vi "_OLS_RunReport_Rev3.vi"() -> ()   [LabVIEW 2024]
uses:
  Control Definitions/Def Results2.ctl
  Control Definitions/Def_ATPStatus.ctl
  Control Definitions/Def_PumpSpeed.ctl
  Control Definitions/Def TestState.ctl
  Control Definitions/DEF_CalConstants.ctl
  Control Definitions/Def PumpCtlRefs.ctl
  Control Definitions/Def CalTable.ctl
  Control Definitions/Def CalCoef.ctl
  Control Definitions/Def_LevelCalCoef.ctl
  Control Definitions/Registry Keys.ctl
  Control Definitions/Global 2.vi
  Control Definitions/Global 1.vi
panel:
  in  "Get File Data":bool=TRUE
  in  "Level PV":dbl(slide)=8.0 scale=8.5..2.0
  out "File Name":string
  out "Root path":path
  out "Numeric":i32
  out "Cal Coef":T1={"Level"={"M"=-0.9990777034816695, "B"=9.617362923679963, "Mc"=-1.0009231479344565, "Bc"=9.626241172397878, "LMe"=7.844}, "Dataq Ch"=[{"B"=-0.34241100677002123, "M"=175.4094780519764}, {"B"=-0.7865736704446391, "M"=174.89102005231038}]}
  in  "Default Cal Table":T3={"Level"={"LSf"=2.6, "LMf"=3.511, "LKf"=6.112, "LMe"=7.844, "LKe"=1.775, "LSe"=8.0}, "DataQ CH"=[{"RqLA"=0.577, "RmLA"=102.9, "RqHA"=5.052, "RmHA"=904.4}, {"RqLA"=0.577, "RmLA"=101.1, "RqHA"=5.116, "RmHA"=903.4}]}
  out "ItemPath":string
  in  "End Prog":bool=TRUE
  out "Test Index Out":i32
  out "PumpCtlRef out":T4
  out "Reg Cal Constants":T5={"Measure High"="", "Laser High"="", "Measure Low"="", "Laser Low"="", "Cal Name"="", "Cal Date"="9/24/2024 9:21:12 AM", "Empty Inches"=8.0, "Full Inches"=2.6, "Valid"=FALSE}
  in  "Skip Pre-Lube":bool=TRUE
  out "TEST State Out":T6
  in  "Pump Speed":T7
  out "Ch B  Sim":dbl=101.0
  out "Ch A  Sim":dbl=200.0
  out "Root Path":path=path "C:/AllenProjects/PWC-OLS"
  out "Time(ms)":dbl=1249.4499999994114
  out "Level":bool=TRUE
  out "DataQ":bool=TRUE
  in  "Check":bool
  out "Laser (raw)":dbl=1.9040000438690186 format="%#_4g"
  out "Results out":T8 {"Resistor" format="%.1f"; "Drain" format="%.3f"; "Fill" format="%.3f"}
  in  "DUT":i16=1
  in  "Pump JOG":bool=TRUE
  in  "Run Test":bool
  in  "Normal":cluster{u32, u32}[](array[cluster])=[{16711680, 1244948}]
  in  "Sim Color":cluster{u32, u32}[](array[cluster])=[{16774656, 1244948}]
  out "Level \nStatus":bool=TRUE
  out "DataQ\nStatus":bool=TRUE
  in  "Level SP":dbl(slide)=8.0 scale=8.5..2.0
  out "Level":dbl=7.715118932422306 format="%.3f"
  in  "Drain":bool
  in  "Fill":bool
  in  "Simulate":bool
  out "TEST NME":string="OLR001--cal"
  out "DataQ Input":T10(graph)={"ChA Ohms"=100.83065830421491, "ChB Ohms"=100.0340857774357, "Laser (raw)"=1.9040000438690186}
  out "Time Stamp":timestamp=timestamp(3810639016.2712703 s since 1904-01-01)
  in  "stop":bool
  out "ChB Ohms":dbl=100.0340857774357 format="%.1f"
  out "ChA Ohms":dbl=100.79497115454612 format="%.1f"
  out "TimeBase":dbl=100.79497115454612 format="%.1f"
  # "Calibration & Scaling Table\n               Tank         Key          Ref\n               Scale        Level        Measure\nEmpty\n\n\nFull"
  # "8.0      1.7752      7.844\n\n2.6      6.112        3.511"
  # "CHA"
  # "CHB"
  # "ATP       Resistance     Fill        Drain"
  # "ATP       Resistance     Fill        Drain"
  # "Simulated Resistor In"
  # "PUMP"
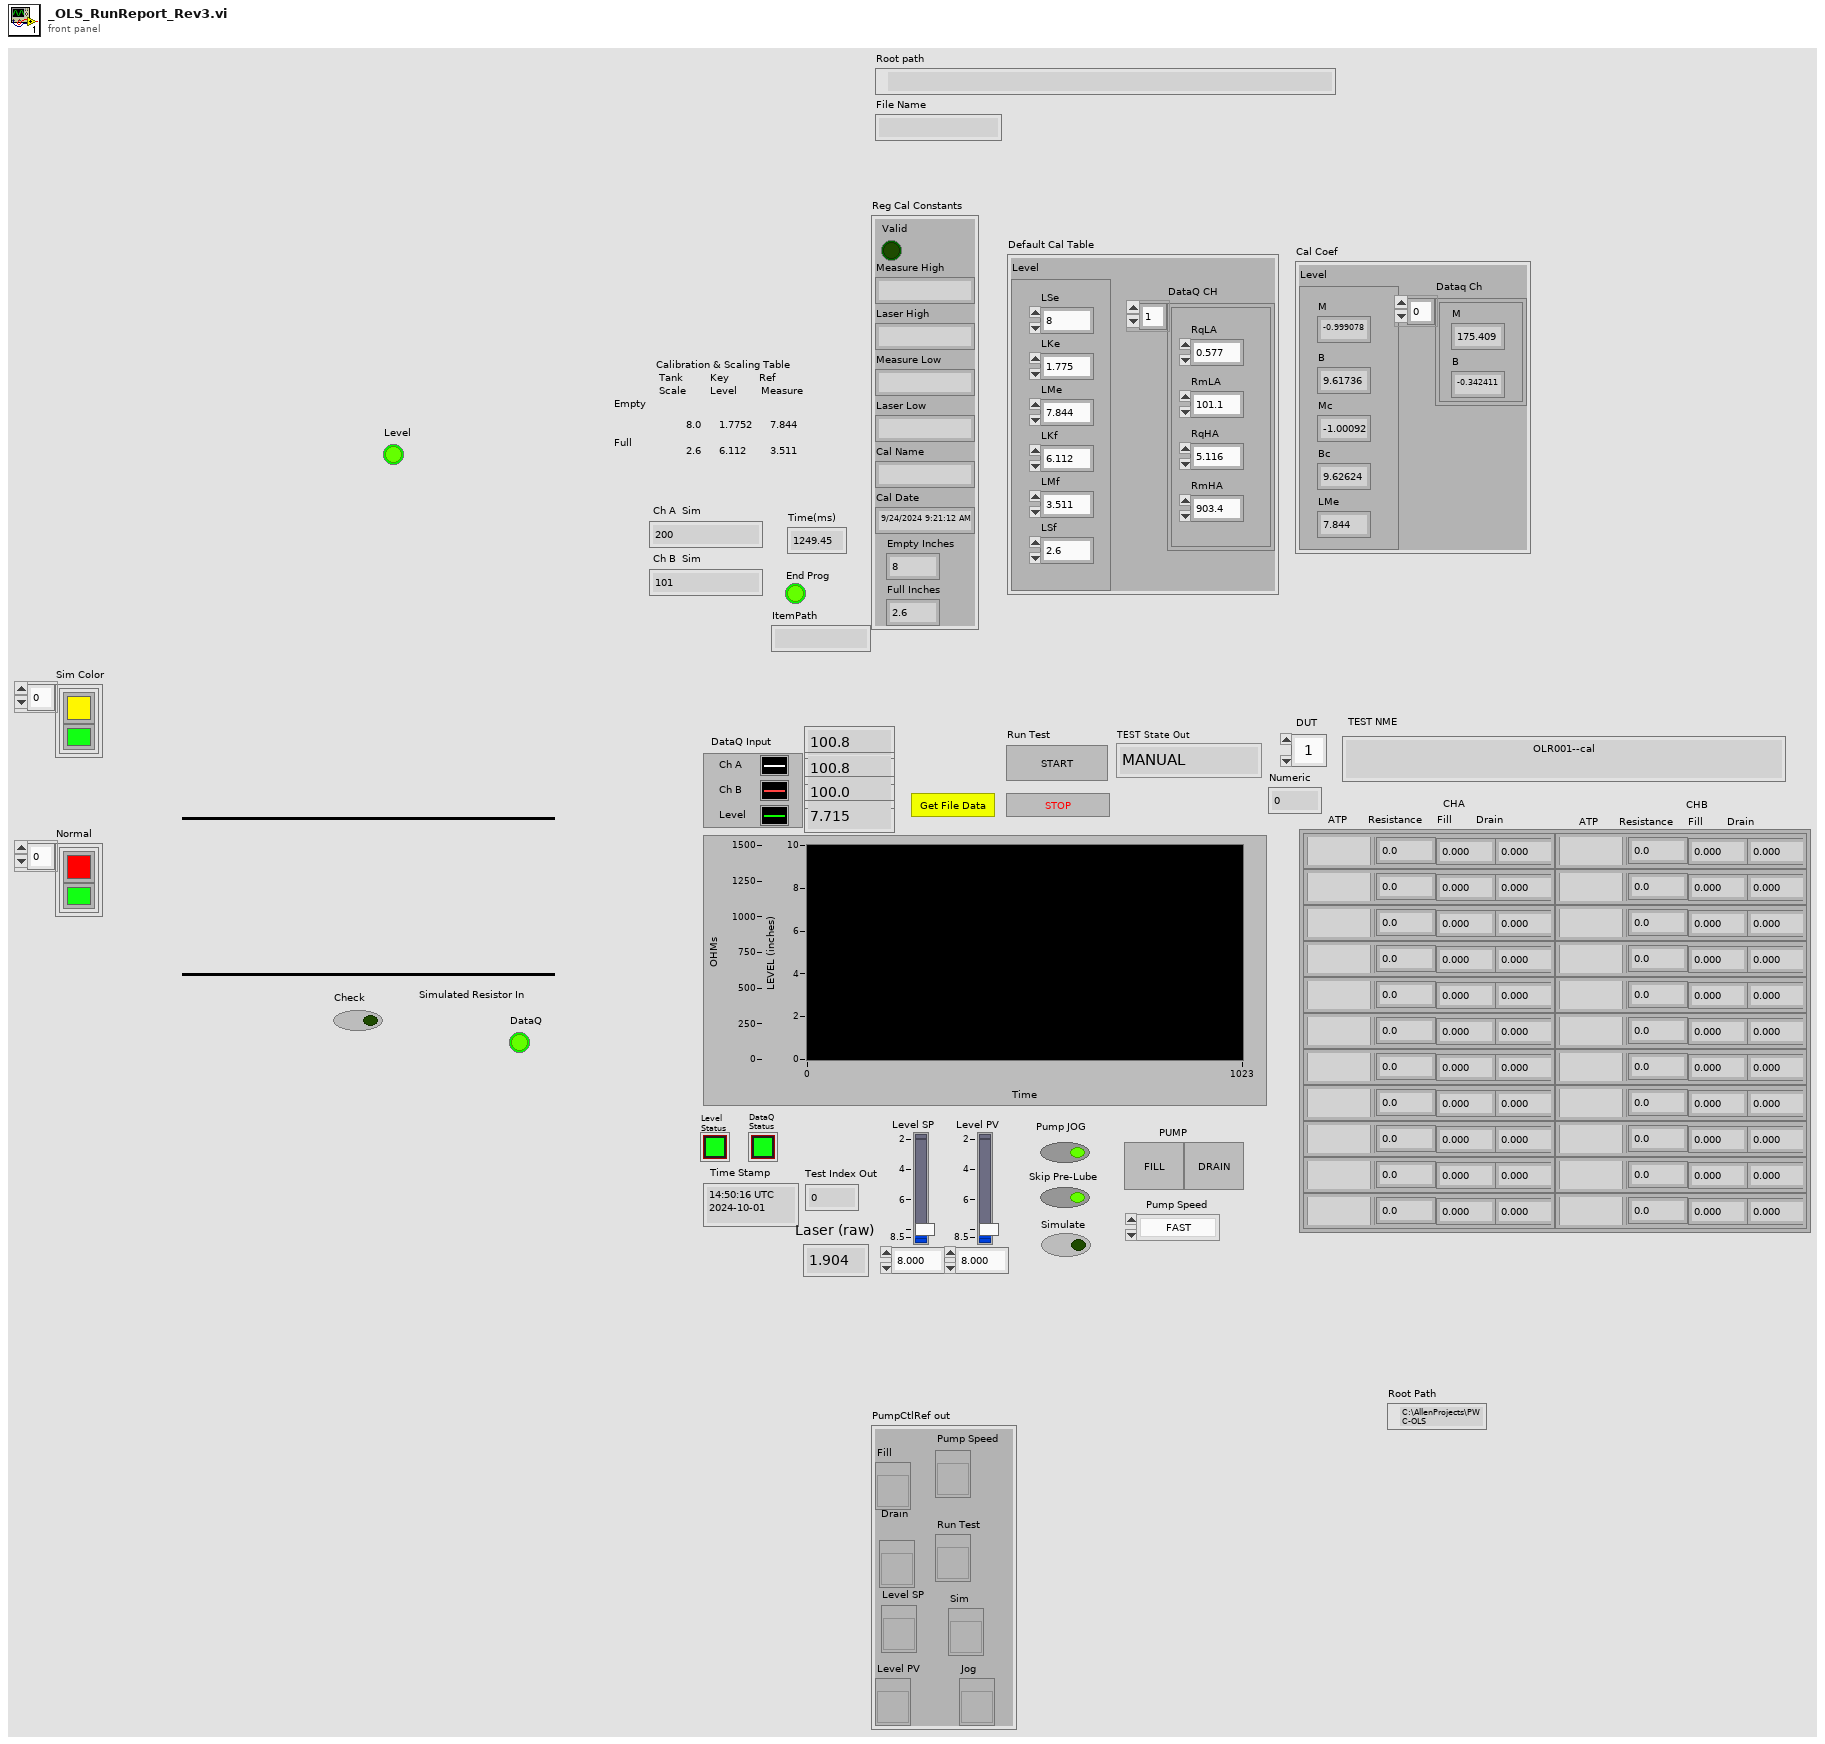
[diagram p1: front panel]
types:
  T1 = typedef "Def CalCoef.ctl" = cluster{"Level":T2, "Dataq Ch":cluster{"B":dbl, "M":dbl}[]}
  T2 = typedef "Def_LevelCalCoef.ctl" = cluster{"M":dbl, "B":dbl, "Mc":dbl, "Bc":dbl, "LMe":dbl}
  T3 = typedef "Def CalTable.ctl" = cluster{"Level":cluster{"LSf":dbl, "LMf":dbl, "LKf":dbl, "LMe":dbl, "LKe":dbl, "LSe":dbl}, "DataQ CH":cluster{"RqLA":dbl, "RmLA":dbl, "RqHA":dbl, "RmHA":dbl}[]}
  T4 = typedef "Def PumpCtlRefs.ctl" = cluster{"Fill ":refnum<vi>, "Drain":refnum<vi>, "Level PV":refnum<vi>, "Pump Speed":refnum<vi>, "Run Test":refnum<vi>, "Sim":refnum<vi>, "Jog":refnum<vi>, "Level SP":refnum<vi>}
  T5 = typedef "DEF_CalConstants.ctl" = cluster{"Measure High":string, "Laser High":string, "Measure Low":string, "Laser Low":string, "Cal Name":string, "Cal Date":string, "Empty Inches":dbl, "Full Inches":dbl, "Valid":bool}
  T6 = typedef "Def TestState.ctl" = enum16{"MANUAL", "Start", "Pre-Fill", "Pre-Fill Measure", "Pre-Drain", "Pre-Drin Measure", "Init-Record", "Load Fill Spec", "Filling Hi", "Wait1", "Record Fill", "Load Drain Spec", "Draining Lo", "Wait2", "Record Drain", "Empty", "Done"}
  T7 = typedef "Def_PumpSpeed.ctl" = enum16{"FAST", "SLOW", "CREEP", "STOP"}
  T8 = typedef "Def Results2.ctl" = cluster{"Fill":dbl, "Drain":dbl, "Status":T9, "Resistor":dbl}[][]
  T9 = typedef "Def_ATPStatus.ctl" = i16
  T10 = cluster{"ChA Ohms":dbl, "ChB Ohms":dbl, "Laser (raw)":dbl}
  T11 = typedef "Registry Keys.ctl" = enum16{"Report Files Key", "Config Files Key"}
  T12 = cluster{"Level \nStatus":refnum<vi>, "DataQ\nStatus":refnum<vi>}
  T13 = typedef "Def FullCfg.ctl" = cluster{"Bench Config":T14, "Test Value Table ":dbl[][], "Table Col Titles":string[][], "cluster":T4, "Bench Status":T15}
  T14 = typedef "Def BenchCfg.ctl" = cluster{"Name":string, cluster{"Step Levels":dbl, "Tolerance":dbl, "Sample Rate":dbl, "Resistor":dbl, "M Level Cal":dbl, "[B Level Cal":dbl, "Max Fill Rate":dbl, "Empty Inches":dbl, "Full Inches":dbl}}
  T15 = typedef "Def Bench Status.ctl" = cluster{"Pump Status":refnum<vi>, "Instrumnet\n Status":refnum<vi>}
  T16 = enum16{"MANUAL", "Start", "Filling", "FULL", "Draining", "EMPTY", "Done"}
  T17 = cluster{"Resistor":dbl, "Fill":dbl, "Drain":dbl, "Status":i16}
  T18 = cluster{"Resistor":dbl, "Fill":dbl, "Drain":dbl, "Status":i16}[][]
  T19 = typedef "DEF_SpecsOut.ctl" = cluster{"aSpecsTable":T20[], "Pump CtlRef In":T4, "TEST State Out":T6, "TEST Index":i32, "Drain!Fill":bool}
  T20 = typedef "Def Spec RNG.ctl" = cluster{"Specs":dbl[], "LUT Status":T21}
  T21 = typedef "Ded LUT_Status.ctl" = cluster{"ChA/!ChB":bool, "Drain/!Fill":bool, "In Range?":bool, "Switch Range?":bool, "Measure R?":bool, "Vaild R?":bool, "Index(n)":i32, "Index(n)-1":i32, "Index Max":i32, "Index(n-1)":i32}
  T22 = typedef "Def Measure.ctl" = cluster{"ChA R":dbl, "ChB R":dbl, "Level PV":dbl}
  T23 = cluster{"Resistor":dbl, "Fill":dbl, "Drain":dbl, "Resistor":dbl}[][]
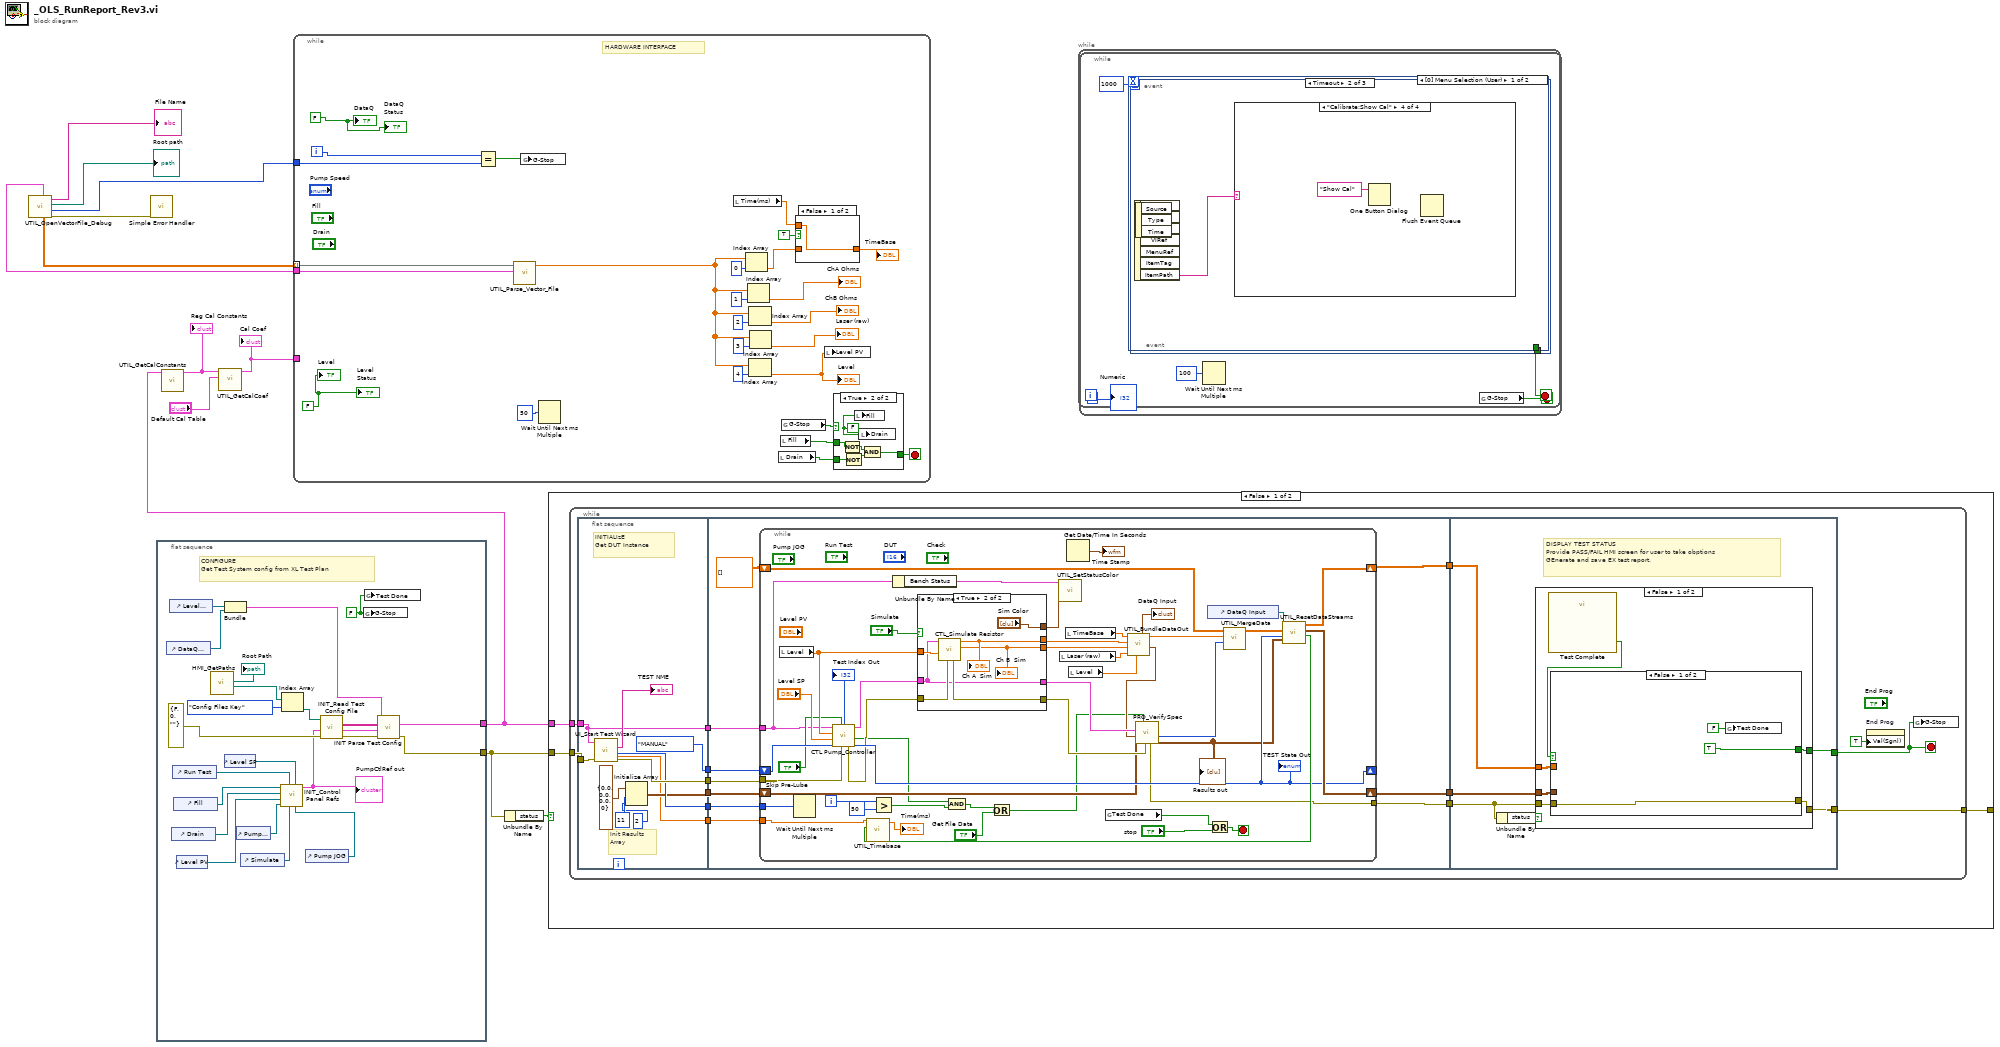
[diagram p0: block diagram]
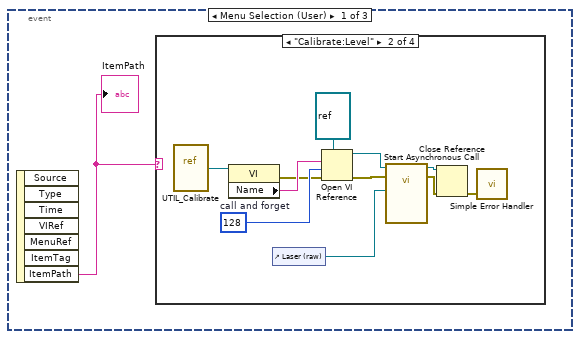
[diagram p2: hidden frame]
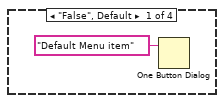
[diagram p3: hidden frame]
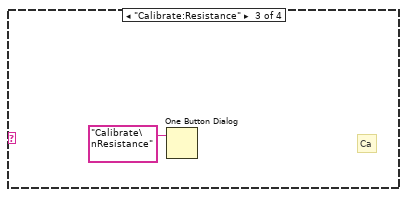
[diagram p4: hidden frame]
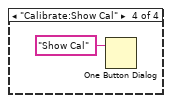
[diagram p5: hidden frame]
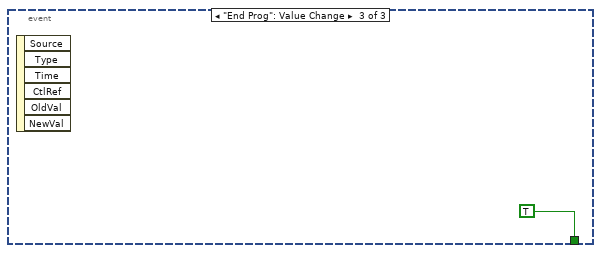
[diagram p6: hidden frame]
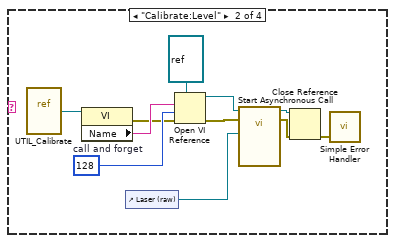
[diagram p8: hidden frame]
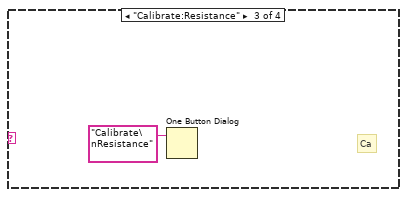
[diagram p9: hidden frame]
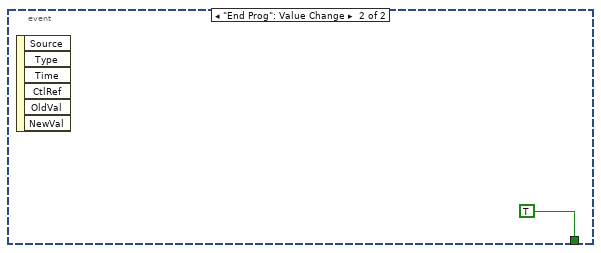
[diagram p10: hidden frame]
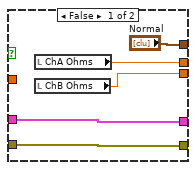
[diagram p11: hidden frame]
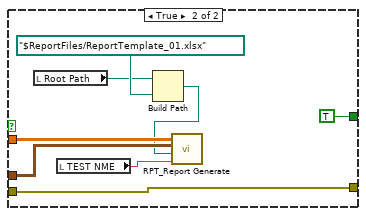
[diagram p12: hidden frame]
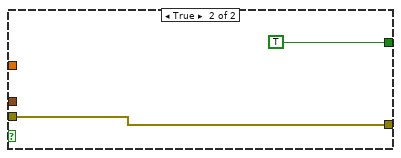
[diagram p13: hidden frame]
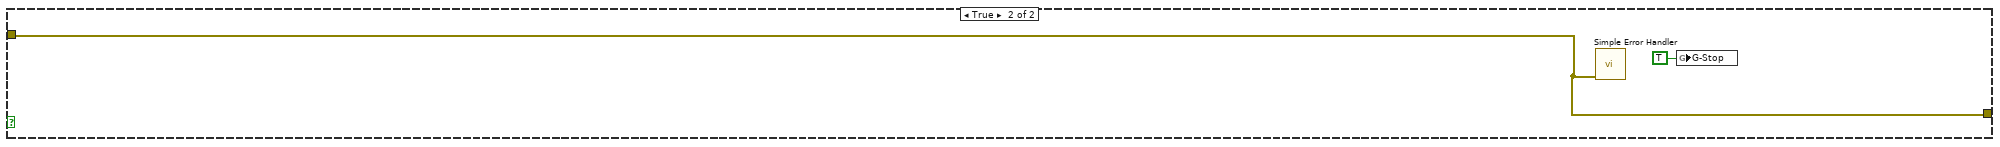
[diagram p14: hidden frame]
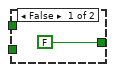
[diagram p16: hidden frame]
diagram:
  n1 = call "UTIL_OpenVectorFile_Debug.vi"() -> ("error out"=w4:errorcluster, "Count"=w1:i32, "path"=→"Root path":path, "File Name"=→"File Name":string, "Data"=w3:dbl[][], "Cal Coef Out"=w2:T1)  [unwired: 6 in]
  n2 = call <vilib>:"Simple Error Handler.vi"("error in (no error)"=w4) -> ()  [unwired: 4 in, 5 out]
  n3 = flat-sequence {
    tunnel: [w32] -> w11
    tunnel: [w25] -> w9
    frame #0 {
      w20 = FALSE ("G-Stop")
      # "CONFIGURE\nGet Test System config from XL Test Plan"
      n4 = control-ref of="DataQ\nStatus"() -> (w22:refnum<vi>)
      n5 = control-ref of="Level \nStatus"() -> (w31:refnum<vi>)
      n6 = control-ref of="Drain"() -> (w33:refnum<vi>)
      n7 = control-ref of="Run Test"() -> (w27:refnum<vi>)
      n8 = control-ref of="Fill"() -> (w28:refnum<vi>)
      n9 = control-ref of="Level PV"() -> (w13:refnum<vi>)
      n10 = call "HMI_GetPaths.vi"() -> ("Default Paths"=w15:path[], "Root Path"=→"Root Path":path)  [unwired: 10 in]
      n11 = Bundle("Level \nStatus"=w31, "DataQ\nStatus"=w22) -> (w30:T12)  [unwired: 1 in]
      n12 = control-ref of="Level SP"() -> (w21:refnum<vi>)
      n13 = control-ref of="Pump Speed"() -> (w17:refnum<vi>)
      n14 = control-ref of="Simulate"() -> (w24:refnum<vi>)
      n15 = Index Array(array=w15, index=Registry_Keys."Config Files Key" ("Reg Key")) -> (element=w14:path)
      n16 = control-ref of="Pump JOG"() -> (w23:refnum<vi>)
      n17 = call "INIT_Control Panel Refs.vi"("Jog"=w23, "Level SP"=w21, "Sim"=w24, "Run Test"=w27, "Pump Speed"=w17, "Level PV"=w13, "Drain"=w33, "Fill"=w28) -> ("PumpCtlRef out"=w18:T4)  [unwired: 3 in]
      "PumpCtlRef out" <- w18
      n18 = call "INIT_Read Test Config File.vi"("error in (no error)"=errorcluster {"status"=FALSE, "code"=0, "source"=""}, "Path"=w14) -> ("error out 2"=w26:errorcluster, "Config\nFile Data"=w29:string[][])  [unwired: 8 in]
      n19 = global write "Global 1.vi" "G-Stop"(w20) -> ()
      n20 = global write "Global 2.vi" "Test Done"(w20) -> ()
      n21 = call "INIT Parse Test Config.vi"("error in (no error)"=w26, "Pump CtlRef In"=w18, "All XL Input"=w29, "Bench Status"=w30) -> ("error out"=w32:errorcluster, "Full Config"=w25:T13)  [unwired: 5 in, 1 out]
    }
  }
  n22 = call "UTIL_GetCalConstants.vi"("Full Config"=w9) -> ("Cal Constants"=w10:T5)  [unwired: 9 in, 1 out]
  "Reg Cal Constants" <- w10
  n23 = call "UTIL_GetCalCoef.vi"("Cal Table"="Default Cal Table", "Cal Constants"=w10) -> ("Cal Coef"=w7:T1)  [unwired: 9 in]
  "Cal Coef" <- w7
  n24 = while {
    tunnel: w7 -> [_]
    tunnel: w3 -> [w55] mode=indexing
    tunnel: w2 -> [w49]
    tunnel: w1 -> [w53]
    i -> [w54]
    stop <- w58 stop-if-true
    w50 = FALSE
    w51 = FALSE
    # "HARDWARE INTERFACE"
    n25 = Equal?(x=w54, y=w53) -> (x = y?=w52:bool)
    n26 = call "UTIL_Parse_Vector_File.vi"("Cal Coef"=w49, "Data IN"=w55) -> ("Data Out"=w43:dbl[])  [unwired: 6 in, 3 out]
    n27 = global write "Global 1.vi" "G-Stop"(w52) -> ()
    n28 = Wait Until Next ms Multiple(millisecond multiple=u32 50) -> ()  [unwired: 1 out]
    n29 = local read "Time(ms)"() -> (w35:dbl)
    n30 = Index Array(array=w43, index=0) -> (element=w38:dbl)
    n31 = Index Array(array=w43, index=1) -> (element=→"ChA Ohms":dbl)
    n32 = Index Array(array=w43, index=2) -> (element=→"ChB Ohms":dbl)
    n33 = Index Array(array=w43, index=4) -> (element=w39:dbl)
    "Level" <- w39
    n34 = Index Array(array=w43, index=3) -> (element=→"Laser (raw)":dbl)
    n35 = local read "Drain"() -> (w56:bool)
    n36 = local read "Fill"() -> (w57:bool)
    n37 = global read "Global 1.vi" "G-Stop"() -> (w59:bool)
    n38 = case shown="False" TRUE {
      tunnel: w38 -> [_ w62]
      tunnel: [w61 w62] -> w37
      tunnel: w35 -> [w61 _]
      frame False {
      }
      frame True {
      }
    }
    "TimeBase" <- w37
    n39 = local write "Level PV"(w39) -> ()
    n40 = case shown="True" w59 {
      tunnel: [FALSE w65] -> w58
      tunnel: w57 -> [_ w67]
      tunnel: w56 -> [_ w64]
      frame False {
      }
      frame True {
        w69 = FALSE
        n41 = Not(x=w67) -> (.not. x?=w68:bool)
        n42 = Not(x=w64) -> (.not. x?=w66:bool)
        n43 = local write "Fill"(w69) -> ()
        n44 = local write "Drain"(w69) -> ()
        n45 = And(x=w68, y=w66) -> (x .and. y?=w65:bool)
      }
    }
    "DataQ\nStatus" <- w50
    "Level \nStatus" <- w51
    "DataQ" <- w50
    "Level" <- w51
  }
  n46 = Unbundle By Name(w11) -> ("status"=w12:bool)
  n47 = case shown="False" w12 {
    tunnel: w11 -> [w72 w192]
    tunnel: w9 -> [w71 _]
    tunnel: [w70 w192] -> _
    frame False {
      n48 = while {
        tunnel: w72 -> [w83]
        tunnel: w71 -> [w81]
        tunnel: [w76] -> w70
        stop <- w74 stop-if-true
        n49 = flat-sequence {
          tunnel: [w95] -> w85
          tunnel: [w96] -> w84
          tunnel: w83 -> [w97]
          tunnel: [w87] -> w82
          tunnel: w81 -> [w87]
          tunnel: [T16."MANUAL" ("TEST STATUS Out")] -> w80
          tunnel: [w90] -> w79
          tunnel: [w89] -> w75
          tunnel: [w101] -> w86
          tunnel: w85 -> [w106]
          tunnel: w84 -> [w107]
          tunnel: w82 -> [w98]
          tunnel: w80 -> [w99]
          tunnel: w79 -> [w105]
          tunnel: [w104] -> w78
          tunnel: [w103] -> w77
          tunnel: w75 -> [w102]
          tunnel: w86 -> [w172]
          tunnel: [w171] -> w74
          tunnel: [w169] -> w76
          tunnel: w78 -> [w168]
          tunnel: w77 -> [w167]
          frame #0 {
            # "Init Results\nArray"
            # "INITIALIzE\nGet DUT Instance"
            n50 = call "UI_Start Test Wizard.vi"("error in (no error)"=w97, "Full Config"=w87) -> ("error out"=w96:errorcluster, "Time Base mS"=w95:i32, "Title"=→"TEST NME":string, "Sample Rate"=w89:dbl)  [unwired: 4 in]
            n51 = Initialize Array(T17 {"Resistor"=0.0, "Fill"=0.0, "Drain"=0.0, "Status"=0} ("Cluster 2"), 11 ("dimension size"), 2 ("dimension size")) -> (w90:T18)
          }
          frame #1 {
            n52 = while {
              tunnel: w106 -> [w152]
              tunnel: w107 -> [w141]
              tunnel: [w129] -> w101
              shift-right: [w135] -> w103
              shift-left: w105 -> [w128]
              tunnel: w102 -> [w140]
              shift-right: [w136] -> w104
              shift-left: dbl[][] [] ("Array") -> [w122]
              shift-right: [w132] -> _
              shift-left: w99 -> [w131]
              tunnel: w98 -> [w112]
              i -> [w139]
              stop <- w149 stop-if-true
              n53 = local read "Level"() -> (w117:dbl)
              n54 = Wait Until Next ms Multiple(millisecond multiple=w152) -> ()  [unwired: 1 out]
              n55 = call "CTL Pump_Controller.vi"("error in (no error)"=w141, "Skip Pre-Lub"="Skip Pre-Lube", "TEST State In"=w131, "Level SP"="Level SP", "Level PV"=w117, "Full Cfg 2"=w112) -> ("TEST State Out"=w132:T6, "Enable"=w113:bool, "Specs Out"=w115:T19, "error out"=w114:errorcluster, "Test Index Out"=→"Test Index Out":i32)  [unwired: 1 in]
              "TEST State Out" <- w132
              n56 = Greater?(x=w139, y=50) -> (0:w137:bool)
              n57 = Unbundle By Name(w112) -> ("Bench Status"=w150:T15)
              n58 = case shown="True" "Simulate" {
                tunnel: w114 -> [w159 w162]
                tunnel: [w159 w165] -> w130
                tunnel: ["Normal" "Sim Color"] -> w151
                tunnel: [w157 w164] -> w144
                tunnel: [w156 w163] -> w143
                tunnel: w115 -> [w155 w160]
                tunnel: w117 -> [_ w161]
                tunnel: [w155 w160] -> w127
                frame False {
                  n59 = local read "ChA Ohms"() -> (w157:dbl)
                  n60 = local read "ChB Ohms"() -> (w156:dbl)
                }
                frame True {
                  n61 = call "CTL_Simulate Resistor.vi"("error in (no error)"=w162, "Level IN"=w161, "Specs IN"=w160) -> ("Ch B  Ohms"=w163:dbl, "Ch A  Ohms"=w164:dbl, "error out"=w165:errorcluster)  [unwired: 6 in]
                  "Ch A  Sim" <- w164
                  "Ch B  Sim" <- w163
                }
              }
              n62 = And(x=w113, y=w137) -> (x .and. y?=w110:bool)
              n63 = Or(x=w110, y="Get File Data") -> (x .or. y?=w109:bool)
              n64 = call "UTIL_SetStatusColor.vi"("Colors [4] in"=w151, "Bench Status"=w150) -> ()  [unwired: 10 in]
              n65 = local read "Laser (raw)"() -> (w145:dbl)
              n66 = local read "TimeBase"() -> (w146:dbl)
              n67 = Get Date/Time In Seconds() -> (seconds since 1Jan1904=→"Time Stamp":timestamp)
              n68 = local read "Level"() -> (w118:dbl)
              n69 = global read "Global 2.vi" "Test Done"() -> (w147:bool)
              n70 = call "UTIL_BundleDataOut.vi"("Level PV"=w118, "Laser (raw)"=w145, "ChB Ohms"=w143, "ChA Ohms"=w144, "Time (ms)"=w146) -> ("Measure"=w126:T22, "Data Out"=w124:dbl[], "Chart Data"=→"DataQ Input":T10)  [unwired: 3 in, 1 out]
              n71 = call "PRO_VerifySpec.vi"("error in (no error)"=w130, "Enable"=w109, "Results in"=w128, "Measure In"=w126, "Specs In"=w127) -> ("Results out"=w125:T8, "Status Code"=w123:i32, "error out"=w129:errorcluster)  [unwired: 4 in]
              "Results out" <- w125
              n72 = control-ref of="DataQ Input"() -> (w119:refnum<vi>)
              n73 = Or(x=w147, y="stop") -> (x .or. y?=w149:bool)
              n74 = call "UTIL_MergeData.vi"("Status Code"=w123, "New Data"=w124, "Data In"=w122) -> ("Data out"=w121:dbl[][])  [unwired: 8 in]
              n75 = call "UTIL_ResetDataStreams.vi"("Results in"=w125, "TEST State Out"=w132, "Data in"=w121, "WaveformChart in"=w119) -> ("Value (Signaling)"=w133:bool, "Results out 2"=w135:T23, "Array"=w136:dbl[][])  [unwired: 5 in]
              n76 = call "UTIL_Timebase.vi"("Reset"=w133, "Sample Rate"=w140) -> ("Time(ms)"=→"Time(ms)":dbl)  [unwired: 9 in]
            }
          }
          frame #2 {
            # "DISPLAY TEST STATUS\nProvide PASS/FAIL HMI screen for user to take obptions\nGEnerate and save EX test report."
            n77 = Unbundle By Name(w172) -> ("status"=w170:bool)
            n78 = case shown="False" w170 {
              tunnel: w172 -> [w176 w190]
              tunnel: [w177 TRUE] -> w171
              tunnel: [w175 w190] -> w169
              tunnel: w168 -> [w174 _]
              tunnel: w167 -> [w173 _]
              frame False {
                n79 = call "Test Complete"() -> ("SAVE"=w178:bool)  [unwired: 18 in, 1 out]
                n80 = case shown="False" w178 {
                  tunnel: [TRUE TRUE] -> w177
                  tunnel: w176 -> [w180 w188]
                  tunnel: [w180 w188] -> w175
                  tunnel: w174 -> [_ w187]
                  tunnel: w173 -> [_ w186]
                  frame False {
                    n81 = global write "Global 2.vi" "Test Done"(FALSE ("Test Done")) -> ()
                  }
                  frame True {
                    n82 = local read "Root Path"() -> (w184:path)
                    n83 = local read "TEST NME"() -> (w182:string)
                    n84 = Build Path(base path=w184, name or relative path=path "$ReportFiles/ReportTemplate_01.xlsx") -> (appended path=w183:path)
                    n85 = call "RPT_Report Generate.vi"("Report Name"=w182, "template"=w183, "Results"=w186, "Wave Data"=w187) -> ()  [unwired: 8 in]
                  }
                }
              }
              frame True {
              }
            }
          }
        }
        n86 = property on="End Prog" class="Bool (strict)"("Val(Sgnl)"=TRUE ("End Prog")) -> ()  [unwired: 2 in, 2 out]
        n87 = global write "Global 1.vi" "G-Stop"(w74) -> ()
      }
    }
    frame True {
      n88 = call <vilib>:"Simple Error Handler.vi"("error in (no error)"=w192) -> ()  [unwired: 4 in, 5 out]
      n89 = global write "Global 1.vi" "G-Stop"(TRUE ("G-Stop")) -> ()
    }
  }
  n90 = while {
    stop <- w194 stop-if-true
    n91 = event shown="[0] Menu Selection (User)" {
      selector: _ -> [_ _]
      dyn-events: _ -> [_ _]
      timeout: _ -> [_ _]
      tunnel: [_ TRUE] -> w194
      event Menu Selection (User) {
        n92 = event-data() -> ("ItemPath"=w195:string)  [unwired: 1 in, 6 out]
        n93 = case shown="\"Calibrate:Show Cal\"" w195 {
          frame "False", Default {
          }
          frame "Calibrate:Level" {
            w206 = 128  # call and forget
            n94 = vi-ref "UTIL_Calibrate.vi"() -> (w199:refnum<vi>)
            n95 = property class="VI"(reference=w199) -> (error out=w197:errorcluster, "Name"=w198:string)  [unwired: 1 in, 1 out]
            n96 = control-ref of="Laser (raw)"() -> (w196:refnum<vi>)
            n97 = Open VI Reference(type specifier VI Refnum (for type only)=refnum<vi> refnum, vi path=w198, options=w206, error in (no error)=w197) -> (vi reference=w204:refnum<vi>, error out=w203:errorcluster)  [unwired: 2 in]
            n98 = call-by-ref "Start Asynchronous Call"(reference=w204, error in=w203, "Digital in"=w196) -> (reference out=w201:refnum<vi>, error out=w202:errorcluster)  [unwired: 10 in, 1 out]
            n99 = Close Reference(reference=w201, error in (no error)=w202) -> (error out=w200:errorcluster)
            n100 = call <vilib>:"Simple Error Handler.vi"("error in (no error)"=w200) -> ()  [unwired: 4 in, 5 out]
          }
          frame "Calibrate:Resistance" {
            # "Ca"
            n101 = One Button Dialog(message="Calibrate\nResistance") -> ()  [unwired: 1 in, 1 out]
          }
          frame "Calibrate:Show Cal" {
            n102 = One Button Dialog(message="Show Cal") -> ()  [unwired: 1 in, 1 out]
          }
        }
      }
      event "End Prog": Value Change {
        n103 = event-data() -> ()  [unwired: 1 in, 6 out]
      }
    }
  }
  n104 = while {
    i -> [w211]
    stop <- w210 stop-if-true
    n105 = event shown="[1] Timeout" {
      selector: _ -> [_ _ _]
      dyn-events: _ -> [_ _ _]
      timeout: 1000 -> [_ _ _]
      tunnel: [_ _ TRUE] -> _
      event Menu Selection (User) {
        n106 = event-data() -> ("ItemPath"=w214:string)  [unwired: 1 in, 6 out]
        "ItemPath" <- w214
        n107 = case shown="\"Calibrate:Level\"" w214 {
          frame "False", Default {
            n108 = One Button Dialog(message="Default Menu item") -> ()  [unwired: 1 in, 1 out]
          }
          frame "Calibrate:Level" {
            w226 = 128  # call and forget
            n109 = vi-ref "UTIL_Calibrate.vi"() -> (w219:refnum<vi>)
            n110 = property class="VI"(reference=w219) -> (error out=w217:errorcluster, "Name"=w218:string)  [unwired: 1 in, 1 out]
            n111 = control-ref of="Laser (raw)"() -> (w216:refnum<vi>)
            n112 = Open VI Reference(type specifier VI Refnum (for type only)=refnum<vi> refnum, vi path=w218, options=w226, error in (no error)=w217) -> (vi reference=w224:refnum<vi>, error out=w223:errorcluster)  [unwired: 2 in]
            n113 = call-by-ref "Start Asynchronous Call"(reference=w224, error in=w223, "Digital in"=w216) -> (reference out=w221:refnum<vi>, error out=w222:errorcluster)  [unwired: 10 in, 1 out]
            n114 = Close Reference(reference=w221, error in (no error)=w222) -> (error out=w220:errorcluster)
            n115 = call <vilib>:"Simple Error Handler.vi"("error in (no error)"=w220) -> ()  [unwired: 4 in, 5 out]
          }
          frame "Calibrate:Resistance" {
            # "Ca"
            n116 = One Button Dialog(message="Calibrate\nResistance") -> ()  [unwired: 1 in, 1 out]
          }
          frame "Calibrate:Show Cal" {
            n117 = One Button Dialog(message="Show Cal") -> ()  [unwired: 1 in, 1 out]
          }
        }
      }
      event Timeout {
        n118 = event-data() -> ()  [unwired: 1 in, 3 out]
        n119 = Flush Event Queue() -> ()  [unwired: 6 in, 3 out]
      }
      event "End Prog": Value Change {
        n120 = event-data() -> ()  [unwired: 1 in, 6 out]
      }
    }
    n121 = Wait Until Next ms Multiple(millisecond multiple=u32 100) -> ()  [unwired: 1 out]
    n122 = global read "Global 1.vi" "G-Stop"() -> (w210:bool)
    "Numeric" <- w211
  }
